vi "Read Return Code.vi"(8 "error in (no error)":errorcluster, 11 "CONNACK in":refnum<class "CONNACK.lvclass">) -> (0 "error out":errorcluster, 2 "Return Code":T1=enum."Server Unavailable", 3 "CONNACK out":refnum<class "CONNACK.lvclass">)   [LabVIEW 2013, in "MQTT_Control_Packets.lvlib" / "CONNACK.lvclass"]
uses:
  CONNACK.lvclass
  Connect Return Code -- enum.ctl
  ControlPacket/ControlPacket.lvclass/ControlPacket.ctl
  ControlPacket/ControlPacket.lvclass
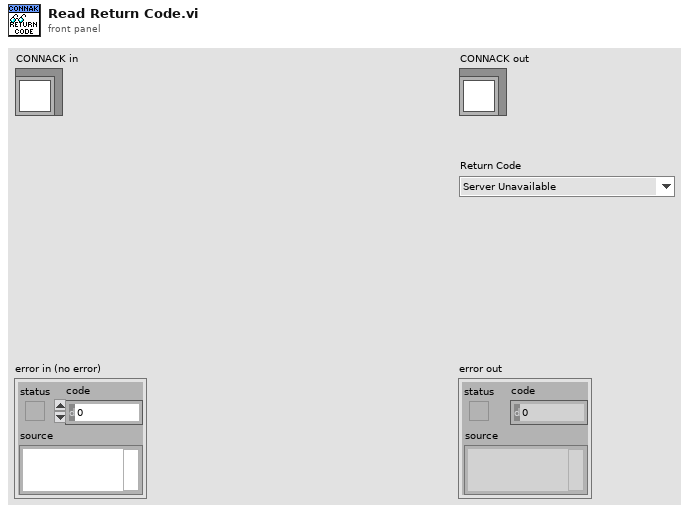
[diagram p1: front panel]
types:
  T1 = typedef "MQTT_Control_Packets.lvlib/CONNACK.lvclass/Connect Return Code -- enum.ctl" = enum16{"Connection accepted", "Unacceptable protocol version", "Identifier Rejected", "Server Unavailable", "Bad Username or Password", "Not Authorized"}
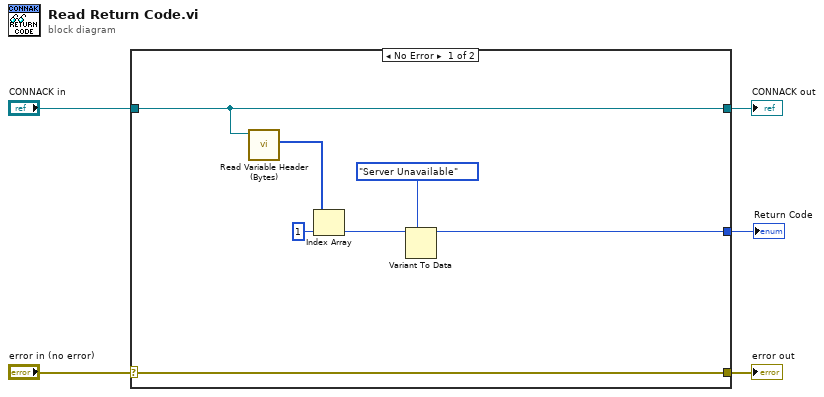
[diagram p0: block diagram]
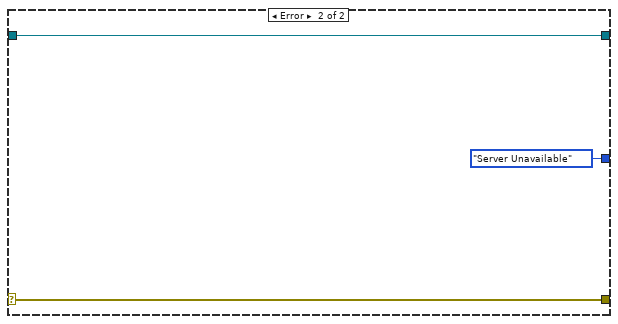
[diagram p2: hidden frame]
diagram:
  n1 = case shown="No Error" "error in (no error)" {
    selector: "error in (no error)" -> [w12 w15]
    tunnel: [w12 w15] -> w4
    tunnel: [w11 w14] -> w2
    tunnel: "CONNACK in" -> [w11 w14]
    tunnel: [w7 Connect_Return_Code_--_enum."Server Unavailable" ("Return Code")] -> w1
    frame No Error {
      n2 = call "Read Variable Header (Bytes).vi"("ControlPacket in"=w11) -> ("Variable Header (Bytes)"=w10:u8[])  [unwired: 9 in, 1 out]
      n3 = Index Array(array=w10, index=1) -> (element=w9:u8)
      n4 = Variant To Data(type=Connect_Return_Code_--_enum."Server Unavailable" ("Return Code"), Variant=w9) -> (data=w7:T1)  [unwired: 1 in, 1 out]
    }
    frame Error {
    }
  }
  "error out" <- w4
  "CONNACK out" <- w2
  "Return Code" <- w1
